vi "set_data_rate.vi"(8 "error in (no error)":errorcluster, 10 "Data rate":u32, 11 "TrajectoryRK110916Throughput in":refnum<class "TrajectoryRK110916Throughput.lvclass">) -> (0 "error out":errorcluster, 3 "TrajectoryRK110916Throughput out":refnum<class "TrajectoryRK110916Throughput.lvclass">)   [LabVIEW 2010, in "TrajectoryRK110916Throughput.lvclass"]
uses:
  TrajectoryRK110916Throughput.lvclass
  TrajectoryRK110916Throughput.lvclass/TrajectoryRK110916Throughput.ctl
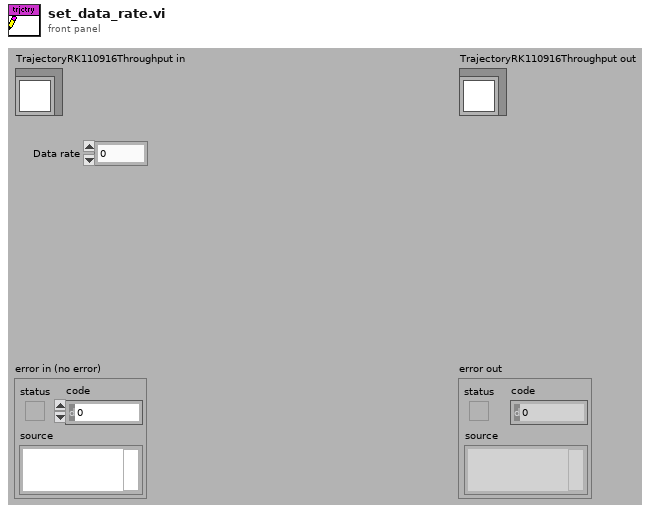
[diagram p1: front panel]
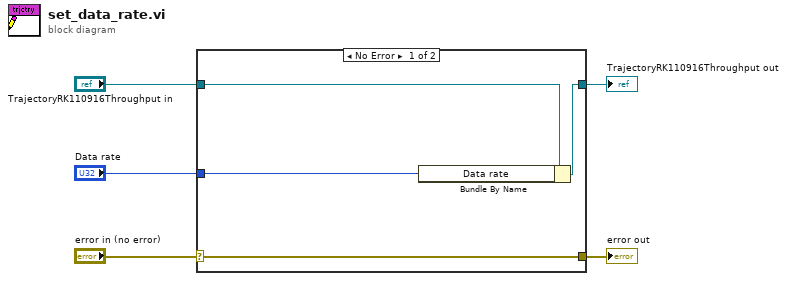
[diagram p0: block diagram]
diagram:
  n1 = case shown="No Error" "error in (no error)" {
    selector: "error in (no error)" -> [w9 w10]
    tunnel: [w9 w10] -> w4
    tunnel: [w7 w11] -> w2
    tunnel: "TrajectoryRK110916Throughput in" -> [w8 w11]
    tunnel: "Data rate" -> [w6 _]
    frame No Error {
      n2 = Bundle By Name(cluster=w8, "Data rate"=w6) -> (w7:refnum<class "TrajectoryRK110916Throughput.lvclass">)
    }
    frame Error {
    }
  }
  "error out" <- w4
  "TrajectoryRK110916Throughput out" <- w2
